vi "总氮启动(子VI).vi"(11 "元素":T1(ring)) -> (0 "error out":T2={"status"=FALSE, "代码"=4, "source"=""} caption="错误输出" {"代码" items=["执行成功"=1, "执行失败，但不知道原因"=2, "命令请求条件错误"=3, "通讯超时"=4, "系统繁忙不能执行"=5, "系统故障"=6, "没有数据"=100]})   [LabVIEW 2016]
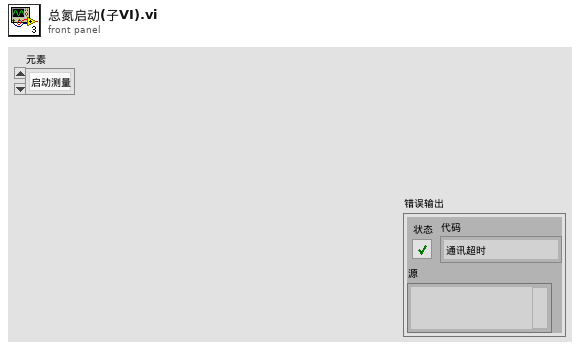
[diagram p1: front panel]
types:
  T1 = enum16{"启动测量", "标样核查", "零点核查", "跨度核查", "空白测试", "平行样测试", "加标回收", "空白校准", "标样校准", "初始化（清洗）", "停止测试", "仪器重启", "校时", "模式设置", "测量间隔设置"}
  T2 = cluster{"status":bool, "代码":u16, "source":string}
  T3 = enum16{"空闲", "水样测试", "标样核查", "零点核查", "跨度核查", "空白测试", "平行样测试", "加标回收", "空白校准", "标样校准", "初始化（清洗）"}
  T4 = cluster{"系统时间":timestamp, "工作状态":u16, "测量模式":enum16{"待机", "连续模式", "周期模式", "定点模式", "受控模式", "手动模式"}, "告警代码":u16, "故障代码":u16, "日志代码":u16, "软件版本":u16, "F0":sgl, "F1":sgl, "F2":sgl, "F3":sgl, "T":sgl, "H":sgl, "id":u16, "flowid":u16, "量程":u16, "总磷控温温度1":sgl, "营养盐控温温度2":sgl, "ADC":sgl}
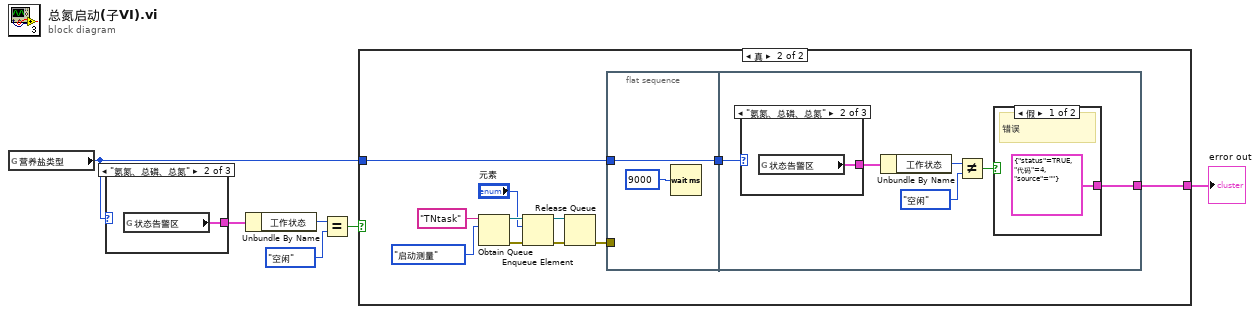
[diagram p0: block diagram]
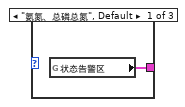
[diagram p2: hidden frame]
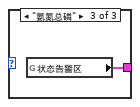
[diagram p3: hidden frame]
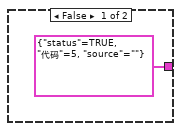
[diagram p4: hidden frame]
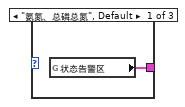
[diagram p5: hidden frame]
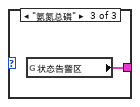
[diagram p6: hidden frame]
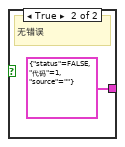
[diagram p7: hidden frame]
diagram:
  n1 = global read "系统设置全局变量.vi" "营养盐类型"() -> (w1:enum16{"氨氮、总磷总氮", "氨氮总磷", "氨氮、总磷、总氮"})
  n2 = case shown="\"氨氮、总磷、总氮\"" w1 {
    tunnel: [w7 w8 w9] -> w4
    frame "氨氮、总磷总氮", Default {
      n3 = global read "VAR总磷总氮全局变量.vi" "状态告警区"() -> (w7:T4)
    }
    frame "氨氮、总磷、总氮" {
      n4 = global read "VAR总磷总氮全局变量.vi" "状态告警区"() -> (w8:T4)
    }
    frame "氨氮总磷" {
      n5 = global read "VAR总磷总氮全局变量.vi" "状态告警区"() -> (w9:T4)
    }
  }
  n6 = Unbundle By Name(w4) -> ("工作状态"=w6:u16)
  n7 = Equal?(x=w6, y=T3."空闲") -> (x = y?=w3:bool)
  n8 = case shown="真" w3 {
    tunnel: [T2 {"status"=TRUE, "代码"=5, "source"=""} ("error out") w18] -> w2
    tunnel: w1 -> [_ w16]
    frame False {
    }
    frame True {
      n9 = Obtain Queue(name (unnamed)="TNtask" ("名称（未命名）"), element data type=T1."启动测量" ("控制命令")) -> (queue out=w13:refnum<queue>, error out=w12:errorcluster)  [unwired: 3 in, 1 out]
      n10 = Enqueue Element(queue=w13, element="元素", error in (no error)=w12) -> (queue out=w21:refnum<queue>, error out=w20:errorcluster)  [unwired: 1 in, 1 out]
      n11 = Release Queue(queue=w21, error in (no error)=w20) -> (error out=w19:errorcluster)  [unwired: 1 in, 2 out]
      n12 = flat-sequence {
        tunnel: w19 -> [_]
        tunnel: [w22] -> w17
        tunnel: w16 -> [w22]
        tunnel: [w29] -> w18
        tunnel: w17 -> [w25]
        frame #0 {
          n13 = Wait (ms)(milliseconds to wait=u32 9000 ("等待时间（毫秒）")) -> ()  [unwired: 1 out]
        }
        frame #1 {
          n14 = case shown="\"氨氮、总磷、总氮\"" w25 {
            tunnel: [w30 w31 w32] -> w24
            frame "氨氮、总磷总氮", Default {
              n15 = global read "VAR总磷总氮全局变量.vi" "状态告警区"() -> (w30:T4)
            }
            frame "氨氮、总磷、总氮" {
              n16 = global read "VAR总磷总氮全局变量.vi" "状态告警区"() -> (w31:T4)
            }
            frame "氨氮总磷" {
              n17 = global read "VAR总磷总氮全局变量.vi" "状态告警区"() -> (w32:T4)
            }
          }
          n18 = Unbundle By Name(w24) -> ("工作状态"=w27:u16)
          n19 = Not Equal?(x=w27, y=T3."空闲") -> (x != y?=w26:bool)
          n20 = case shown="假" w26 {
            tunnel: [T2 {"status"=TRUE, "代码"=4, "source"=""} ("error out") T2 {"status"=FALSE, "代码"=1, "source"=""} ("error out")] -> w29
            frame False {
              # "错误"
            }
            frame True {
              # "无错误"
            }
          }
        }
      }
    }
  }
  "error out" <- w2
